vi "Build.vi"(8 "error in (no error)":errorcluster, 11 "CI Project in":refnum<class "CI Project.lvclass">) -> (0 "error out":errorcluster, 2 "Log Text":string, 3 "CI Project out":refnum<class "CI Project.lvclass">)   [LabVIEW 2014, in "CI Project.lvclass"]
uses:
  CI Project.lvclass
  CI Project.lvclass/CI Project.ctl
  Build Job/Build Job.lvclass/Build Job.ctl
  Build Job/Read Build Name.vi
  Folder Creation/Folder Creation.lvclass
  Build Job/Build Job.lvclass
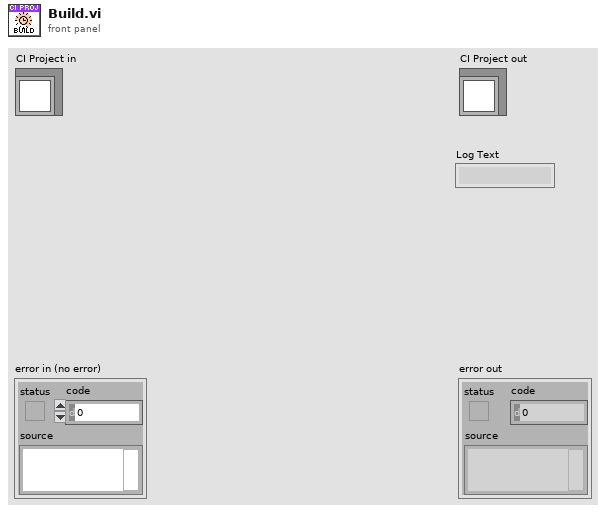
[diagram p1: front panel]
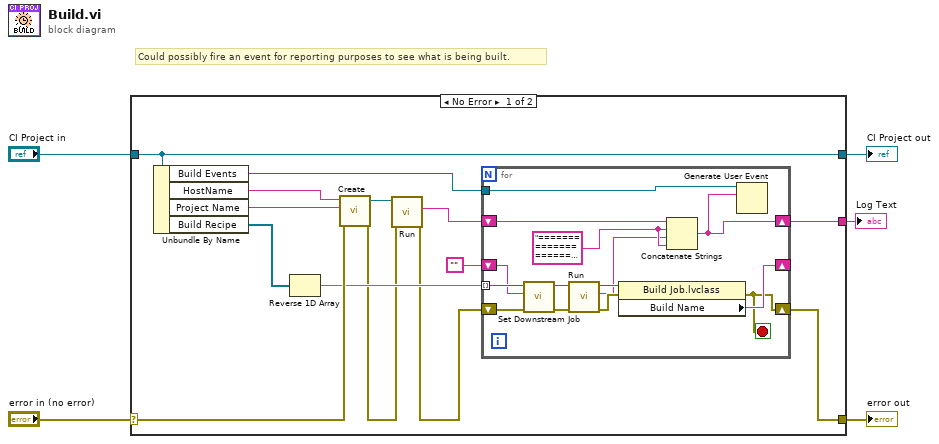
[diagram p0: block diagram]
diagram:
  # "Could possibly fire an event for reporting purposes to see what is being built."
  n1 = case shown="No Error" "error in (no error)" {
    selector: "error in (no error)" -> [w16 w35]
    tunnel: [w9 w35] -> w4
    tunnel: [w19 w34] -> w2
    tunnel: "CI Project in" -> [w19 w34]
    tunnel: [w7 _] -> w1
    frame No Error {
      n2 = Unbundle By Name(w19) -> ("Build Events"=w6:refnum<user-event>, "HostName"=w18:string, "Project Name"=w17:string, "Build Recipe"=w15:refnum<class "Build Job.lvclass">[])
      n3 = Reverse 1D Array(array=w15) -> (reversed array=w14:refnum<class "Build Job.lvclass">[])
      n4 = call "Create.vi"("error in (no error)"=w16, "Folder Name"=w17, "Hostname"=w18) -> ("error out"=w12:errorcluster, "Folder Creation out"=w13:refnum<class "Folder Creation.lvclass">)  [unwired: 7 in]
      n5 = call-dynamic "Run.vi"("error in (no error)"=w12, "Project in"=w13) -> ("error out"=w10:errorcluster, "Text"=w8:string)  [unwired: 7 in, 1 out]
      n6 = for {
        tunnel: w14 -> [w33] mode=indexing
        shift-right: [w27] -> _
        shift-left: "" -> [w31]
        shift-right: [w24] -> w9
        shift-left: w10 -> [w29]
        shift-right: [w20] -> w7
        shift-left: w8 -> [w25]
        tunnel: w6 -> [w23]
        stop <- w24 stop-if-true
        w22 = "===========================================================================\n===========================================================================\n" ("string")
        n7 = call "Set Downstream Job.vi"("error in (no error)"=w29, "Downstream Job"=w31, "Build Job in"=w33) -> ("error out"=w30:errorcluster, "Build Job out"=w32:refnum<class "Build Job.lvclass">)  [unwired: 7 in]
        n8 = call-dynamic "Run.vi"("error in (no error)"=w30, "Project in"=w32) -> ("error out"=w26:errorcluster, "Text"=w21:string, "Project out"=w28:refnum<class "Build Job.lvclass">)  [unwired: 7 in]
        n9 = property class="Build Job.lvclass"(reference=w28, error in=w26) -> (error out=w24:errorcluster, "Build Name"=w27:string)  [unwired: 1 out]
        n10 = Concatenate Strings(w25, w22, w21, w22) -> (w20:string)
        n11 = Generate User Event(user event=w23, event data cluster=w20) -> ()  [unwired: 2 in, 2 out]
      }
    }
    frame Error {
    }
  }
  "error out" <- w4
  "CI Project out" <- w2
  "Log Text" <- w1
